vi "aod_calc_zoom.vi"(8 "FPGA parameters in":T2 {"AOD center frequ. (Hz)_y" format="%.14g"; "AOD half bandwidth_y" format="%.14g"; "AOD Bandwidth_y (Hz)" format="%_6f"; "AOD center frequ. (Hz)_x" format="%.14g"; "cos Phi" format="%.35g"; "sin Phi" format="%.35g"; "AOD_Scale_Factor (1/Zoom)" format="%.35g"; "AOD half bandwidth_x" format="%.14g"; "AOD Bandwidth_x (Hz)" format="%_6f"}, 9 "scan points cluster in":T1, 10 "channel selector in":enum16{"x-channel", "y-channel"}(ring), 11 "point bandwidth":fxp<+,36,32> format="%.29g") -> (0 "FPGA parameters out":T2 {"AOD center frequ. (Hz)_y" format="%.14g"; "AOD half bandwidth_y" format="%.14g"; "AOD Bandwidth_y (Hz)" format="%_6f"; "AOD center frequ. (Hz)_x" format="%.14g"; "cos Phi" format="%.35g"; "sin Phi" format="%.35g"; "AOD_Scale_Factor (1/Zoom)" format="%.35g"; "AOD half bandwidth_x" format="%.14g"; "AOD Bandwidth_x (Hz)" format="%_6f"}, 3 "scaled output":fxp<+/-,36,32> format="%.14g")   [LabVIEW 2010]
uses:
  FPGA_parameters_cluster.ctl
  scan_points_cluster.ctl
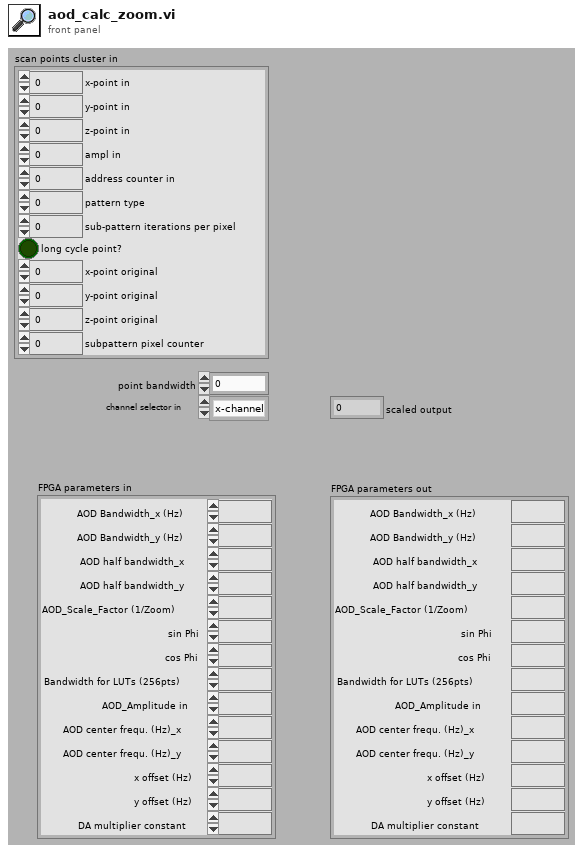
[diagram p1: front panel]
types:
  T1 = typedef "scan_points_cluster.ctl" = cluster{"x-point in":i32, "y-point in":i32, "z-point in":i32, "ampl in":u16, "address counter in":i32, "pattern type":i8, "sub-pattern iterations per pixel":u32, "long cycle point?":bool, "x-point original":i32, "y-point original":i32, "z-point original":i32, "subpattern pixel counter":u32}
  T2 = typedef "FPGA_parameters_cluster.ctl" = cluster{"AOD Bandwidth_x (Hz)":fxp<+,36,32>, "AOD Bandwidth_y (Hz)":fxp<+,36,32>, "AOD half bandwidth_x":fxp<+,36,32>, "AOD half bandwidth_y":fxp<+,36,32>, "AOD_Scale_Factor (1/Zoom)":fxp<+,36,2>, "sin Phi":fxp<+/-,36,2>, "cos Phi":fxp<+/-,36,2>, "Bandwidth for LUTs (256pts)":fxp<+,36,0>, "AOD_Amplitude in":u16, "AOD center frequ. (Hz)_x":fxp<+,36,32>, "AOD center frequ. (Hz)_y":fxp<+,36,32>, "x offset (Hz)":fxp<+/-,36,32>, "y offset (Hz)":fxp<+/-,36,32>, "DA multiplier constant":fxp<+,64,4>}
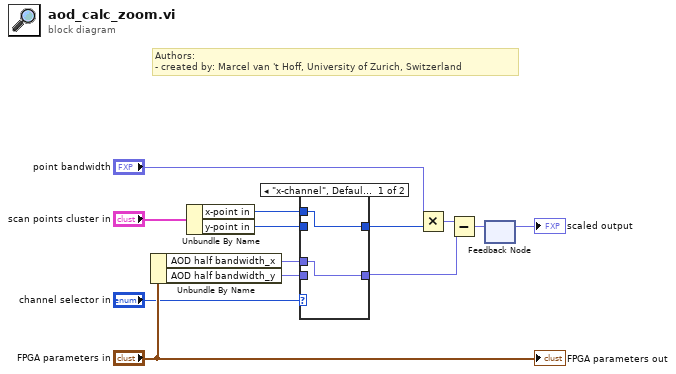
[diagram p0: block diagram]
diagram:
  # "Authors: \n- created by: Marcel van 't Hoff, University of Zurich, Switzerland"
  n1 = Unbundle By Name("FPGA parameters in") -> ("AOD half bandwidth_x"=w9:fxp<+,36,32>, "AOD half bandwidth_y"=w8:fxp<+,36,32>)
  n2 = Unbundle By Name("scan points cluster in") -> ("x-point in"=w6:i32, "y-point in"=w5:i32)
  n3 = case shown="\"x-channel\", Default" "channel selector in" {
    tunnel: [w15 w17] -> w2
    tunnel: w9 -> [w15 _]
    tunnel: w8 -> [_ w17]
    tunnel: w6 -> [w14 _]
    tunnel: w5 -> [_ w16]
    tunnel: [w14 w16] -> w1
    frame "x-channel", Default {
    }
    frame "y-channel" {
    }
  }
  n4 = Multiply(x="point bandwidth", y=w1) -> (x*y=w3:fxp<+,36,32>)
  n5 = Subtract(x=w3, y=w2) -> (x-y=w13:fxp<+/-,36,32>)
  n6 = feedback-in #1(w13) -> ()
  n7 = feedback #1() -> (→"scaled output":fxp<+/-,36,32>)  [unwired: 1 out]
  "FPGA parameters out" <- "FPGA parameters in"
